vi "表格上色.vi"(7 "同色行数":i32, 8 "颜色":cluster{"偶数行颜色盒":u32, "奇数行颜色盒":u32}={"偶数行颜色盒"=16763272, "奇数行颜色盒"=12439011}, 9 "行列总数":cluster{"列总数":i32, "行总数":i32}, 10 "起始行列":cluster{"行":i32, "列":i32}, 11 "引用":refnum<vi>) -> ()   [LabVIEW 2014, in "表格.lvlib" / "表格上色.lvlib"]
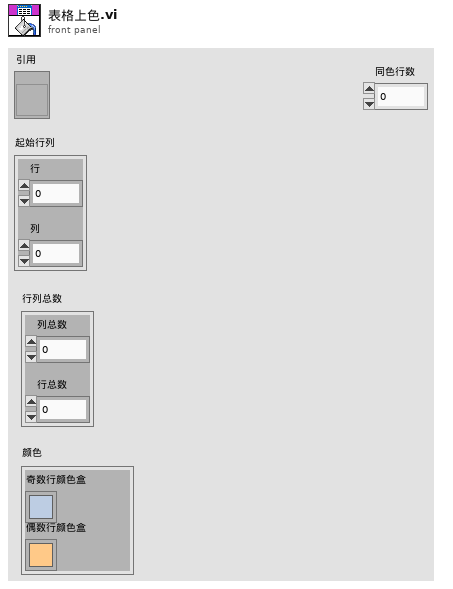
[diagram p1: front panel]
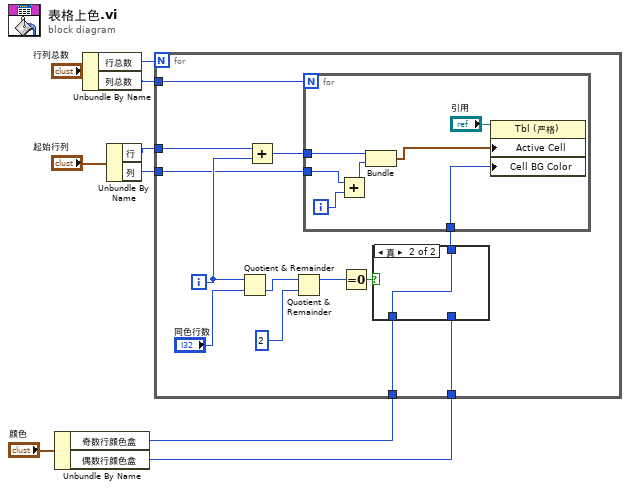
[diagram p0: block diagram]
diagram:
  n1 = Unbundle By Name("颜色") -> ("奇数行颜色盒"=w5:u32, "偶数行颜色盒"=w4:u32)
  n2 = Unbundle By Name("行列总数") -> ("行总数"=w8:i32, "列总数"=w7:i32)
  n3 = Unbundle By Name("起始行列") -> ("行"=w2:i32, "列"=w1:i32)
  n4 = for {
    N: w8 -> [_]
    tunnel: w7 -> [w16]
    tunnel: w5 -> [w15]
    tunnel: w4 -> [w14]
    tunnel: w2 -> [w12]
    tunnel: w1 -> [w10]
    i -> [w13]
    n5 = Quotient & Remainder(x=w13, y="同色行数") -> (floor(x/y)=w19:i32)  [unwired: 1 out]
    n6 = Add(x=w12, y=w13) -> (x+y=w11:i32)
    n7 = Quotient & Remainder(x=w19, y=2) -> (x-y*floor(x/y)=w17:i32)  [unwired: 1 out]
    n8 = Equal To 0?(x=w17) -> (x = 0?=w22:bool)
    n9 = case shown="真" w22 {
      tunnel: [w23 w24] -> w21
      tunnel: w15 -> [_ w24]
      tunnel: w14 -> [w23 _]
      frame False {
      }
      frame True {
      }
    }
    n10 = for {
      N: w16 -> [_]
      tunnel: w11 -> [w31]
      tunnel: w21 -> [w29]
      tunnel: w10 -> [w26]
      i -> [w27]
      n11 = Add(x=w26, y=w27) -> (x+y=w25:i32)
      n12 = Bundle(w31, w25) -> (w30:cluster{i32, i32})  [unwired: 1 in]
      n13 = property on="属性节点" class="Tbl (严格)"(reference="引用", "Active Cell"=w30, "Cell BG Color"=w29) -> ()  [unwired: 1 in, 2 out]
    }
  }
